vi "Auto Match.vi"() -> ()   [LabVIEW 2020]
panel:
  out "Number of Iterations":i32
  out "Current Number":u32 format="%#.0f"
  in  "Number to Match":u32=50 max=1000 step=1
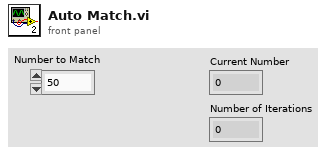
[diagram p1: front panel]
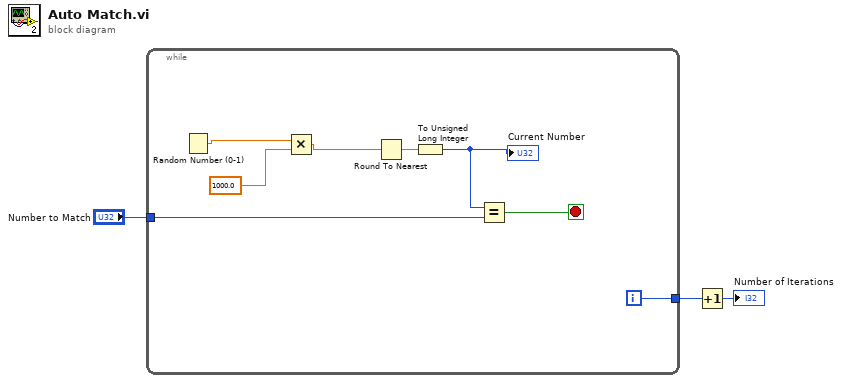
[diagram p0: block diagram]
diagram:
  n1 = while {
    tunnel: "Number to Match" -> [w8]
    tunnel: [w7] -> w1
    i -> [w7]
    stop <- w6 stop-if-true
    n2 = Random Number (0-1)() -> (number: 0 to 1=w11:dbl)
    n3 = Multiply(x=w11, y=1000.0) -> (x*y=w9:dbl)
    n4 = Round To Nearest(number=w9) -> (nearest integer value=w5:dbl)
    n5 = To Unsigned Long Integer(number=w5) -> (unsigned 32bit integer=w4:u32)
    "Current Number" <- w4
    n6 = Equal?(x=w4, y=w8) -> (x = y?=w6:bool)
  }
  n7 = Increment(x=w1) -> (x+1=→"Number of Iterations":i32)
